vi "Coord window-Clear filename ind.vi"(8 "error in (no error)":errorcluster) -> (0 "error out":errorcluster)   [LabVIEW 2017]
uses:
  Globals/Coord window-Globals.vi
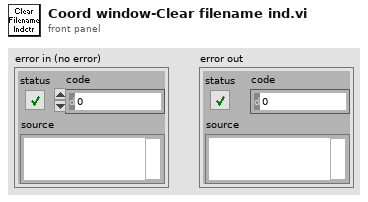
[diagram p1: front panel]
types:
  T1 = typedef "Coordinate list window refs.ctl" = cluster{"Window Name (i.e. Key)":string, "menu reference":refnum<k9>, "VI's reference":refnum<vi>, "Pane 1":refnum<vi>, "Pane 2":refnum<vi>, "Coord Listbox":refnum<vi>, "File name":refnum<vi>, "Picture Map":refnum<vi>, "Stage XYZ Position ind.":refnum<vi>}
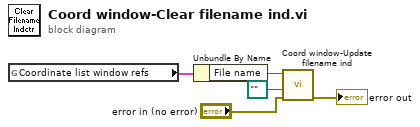
[diagram p0: block diagram]
diagram:
  n1 = global read "Coord window-Globals.vi" "Coordinate list window refs"() -> (w2:T1)
  n2 = Unbundle By Name(w2) -> ("File name"=w1:refnum<vi>)
  n3 = call "Coord window-Update filename ind.vi"("error in (no error)"="error in (no error)", "File path"=path "", "File name indicator ref"=w1) -> ("error out"=→"error out":errorcluster)  [unwired: 8 in]
